vi "Replace Jokers.vi"(11 "Hand":string) -> (3 "Possible Hands":string[](array[string]))   [LabVIEW 2021]
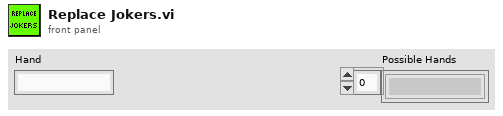
[diagram p1: front panel]
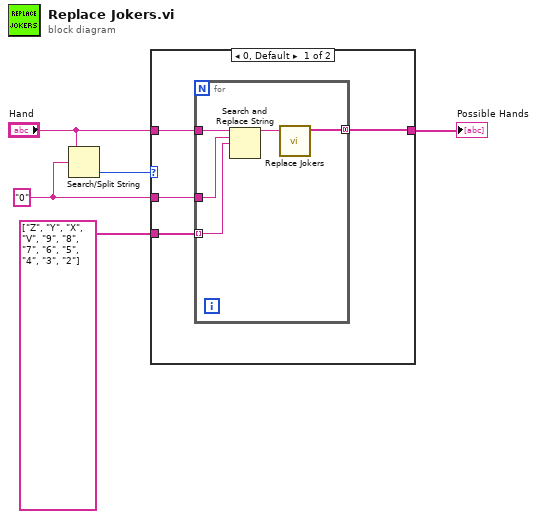
[diagram p0: block diagram]
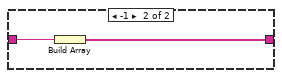
[diagram p2: hidden frame]
diagram:
  w3 = "0"
  n1 = Search/Split String(string="Hand", search string/char (-)=w3) -> (offset of match=w5:i32)  [unwired: 1 in, 2 out]
  n2 = case shown="0, Default" w5 {
    tunnel: "Hand" -> [w9 w16]
    tunnel: [w6 w15] -> w1
    tunnel: w3 -> [w8 _]
    tunnel: string[] ["Z", "Y", "X", "V", "9", "8", "7", "6", "5", "4", "3", "2"] -> [w7 _]
    frame 0, Default {
      n3 = for {
        tunnel: w9 -> [w14]
        tunnel: w8 -> [w13]
        tunnel: w7 -> [w12] mode=indexing
        tunnel: [w10] -> w6 mode=concatenating
        n4 = Search and Replace String(input string=w14, search string=w13, replace string=w12) -> (result string=w11:string)  [unwired: 5 in, 3 out]
        n5 = call "Replace Jokers.vi"("Hand"=w11) -> ("Possible Hands"=w10:string[])  [unwired: 10 in]
      }
    }
    frame -1 {
      n6 = Build Array(w16) -> (w15:string[])
    }
  }
  "Possible Hands" <- w1
